vi "2_VisualizeModulePositioning.vi"(0 "Placement Monitor":T2(plugin-control), 1 "Calibrated positions of fiducials [mm]":dbl[][](array[numeric])=[[-675.4228165149058, -196.82430550413875, -11.55], [-579.8428201474238, -196.8506568257386, -11.55], [-579.816468825824, -101.27066045825673, -11.55], [-675.3964651933059, -101.24430913665685, -11.55], [-577.422820239396, -196.8513240176017, -11.55], [-481.84282387191405, -196.87767533920157, -11.55], [-481.8164725503142, -101.29767897171968, -11.55], [-577.396468917796, -101.2713276501198, -11.55], [-479.42282396388623, -196.87834253106465, -11.55], [-383.8428275964043, -196.90469385266454, -11.55], [-383.81647627480436, -101.32469748518264, -11.55], [-479.3964726422863, -101.29834616358275, -11.55], [-381.42282768837646, -196.90536104452758, -11.55], [-285.8428313208945, -196.93171236612747, -11.55], [-285.8164799992946, -101.35171599864559, -11.55], [-381.39647636677654, -101.3253646770457, -11.55], [-283.4228314128667, -196.93237955799054, -11.55], [-187.84283504538473, -196.95873087959043, -11.55], [-187.8164837237848, -101.37873451210854, -11.55], [-283.39648009126677, -101.35238319050865, -11.55], [-185.42283513735697, -196.9593980714535, -11.55], [-89.84283876987502, -196.98574939305337, -11.55], [-89.81648744827521, -101.40575302557149, -11.55], [-185.39648381575705, -101.3794017039716, -11.55], [-87.42283886184703, -196.98641658491644, -11.55], [8.157157505634814, -197.01276790651633, -11.55], [8.183508827234618, -101.43277153903443, -11.55], [-87.39648754024722, -101.40642021743454, -11.55], [10.57715741366269, -197.01343509837938, -11.55], [106.15715378114453, -197.0397864199793, -11.55], [106.18350510274433, -101.45979005249738, -11.55], [10.603508735262494, -101.4334387308975, -11.55], [108.57715368917252, -197.04045361184234, -11.55], [204.15715005665436, -197.06680493344223, -11.55], [204.18350137825416, -101.48680856596033, -11.55], [108.60350501077232, -101.46045724436046, -11.55], [206.57714996468223, -197.0674721253053, -11.55], [302.1571463321641, -197.09382344690516, -11.55], [302.1834976537639, -101.5138270794233, -11.55], [206.60350128628204, -101.4874757578234, -11.55], [304.57714624019206, -197.09449063876826, -11.55], [400.1571426076739, -197.12084196036813, -11.55], [400.1834939292737, -101.54084559288623, -11.55], [304.60349756179187, -101.51449427128635, -11.55], [402.5771425157018, -197.1215091522312, -11.55], [498.15713888318373, -197.1478604738311, -11.55], [498.18349020478354, -101.56786410634919, -11.55], [402.6034938373016, -101.5415127847493, -11.55], [500.5771387912116, -197.14852766569413, -11.55], [596.1571351586933, -197.17487898729405, -11.55], [596.1834864802931, -101.59488261981214, -11.55], [500.6034901128114, -101.56853129821225, -11.55]], 2 "XYZ .NET Refnum in":refnum<k24>, 3 "Axis Speeds":T5={"X [mm/s]"=25.0, "Y [mm/s]"=12.5, "Z [mm/s]"=5.0}, 4 "Module fiducial marker":T3(ring)=enum."[None]", 5 "N modules":i32=13, 7 "error in (no error)":errorcluster, 8 "Templates path":path=path "C:/Users/Aerotech/Documents/BNL_ThermomechanicalStave", 9 "Calibration [um/pix]":dbl=0.25, 10 "Current Build Phase":refnum<vi>, 12 "Module #":refnum<vi>, 13 "Placement tolerance [um]":dbl=10.0, 16 "Module Report":refnum<vi>) -> (22 "XYZ .NET Refnum out":refnum<k24>, 27 "error out":errorcluster)   [LabVIEW 2016]
uses:
  C:/Users/sciollalab/Documents/Brandeis-BNL/LabVIEW_Codes/BNL_ThermomechanicalStave/AerotechLibraries/Bin/Aerotech.A3200.dll
  AerotechLibraries/Bin/Aerotech.A3200.dll
  <vilib>/vision/NI_Vision_Development_Module.lvlib
panel:
  out "Offset interpreter":T1
  in  "Tab Control":enum32{"Fiducial marker", "Error reporting"}(tab)
  out "Fiducial Template":T2(plugin-control)
  out "Y offset":sgl
  out "X offset":sgl
  out "Current Stage Position":T4
  in  "Module placement loop stop":bool
  out "Module Progress Report":T6(array[cluster])
  # "VISUALIZE MODULE PLACEMENT Brandeis University - Brookhaven National Laboratory * ATLAS Phase II Inner Tracker Upgrade"
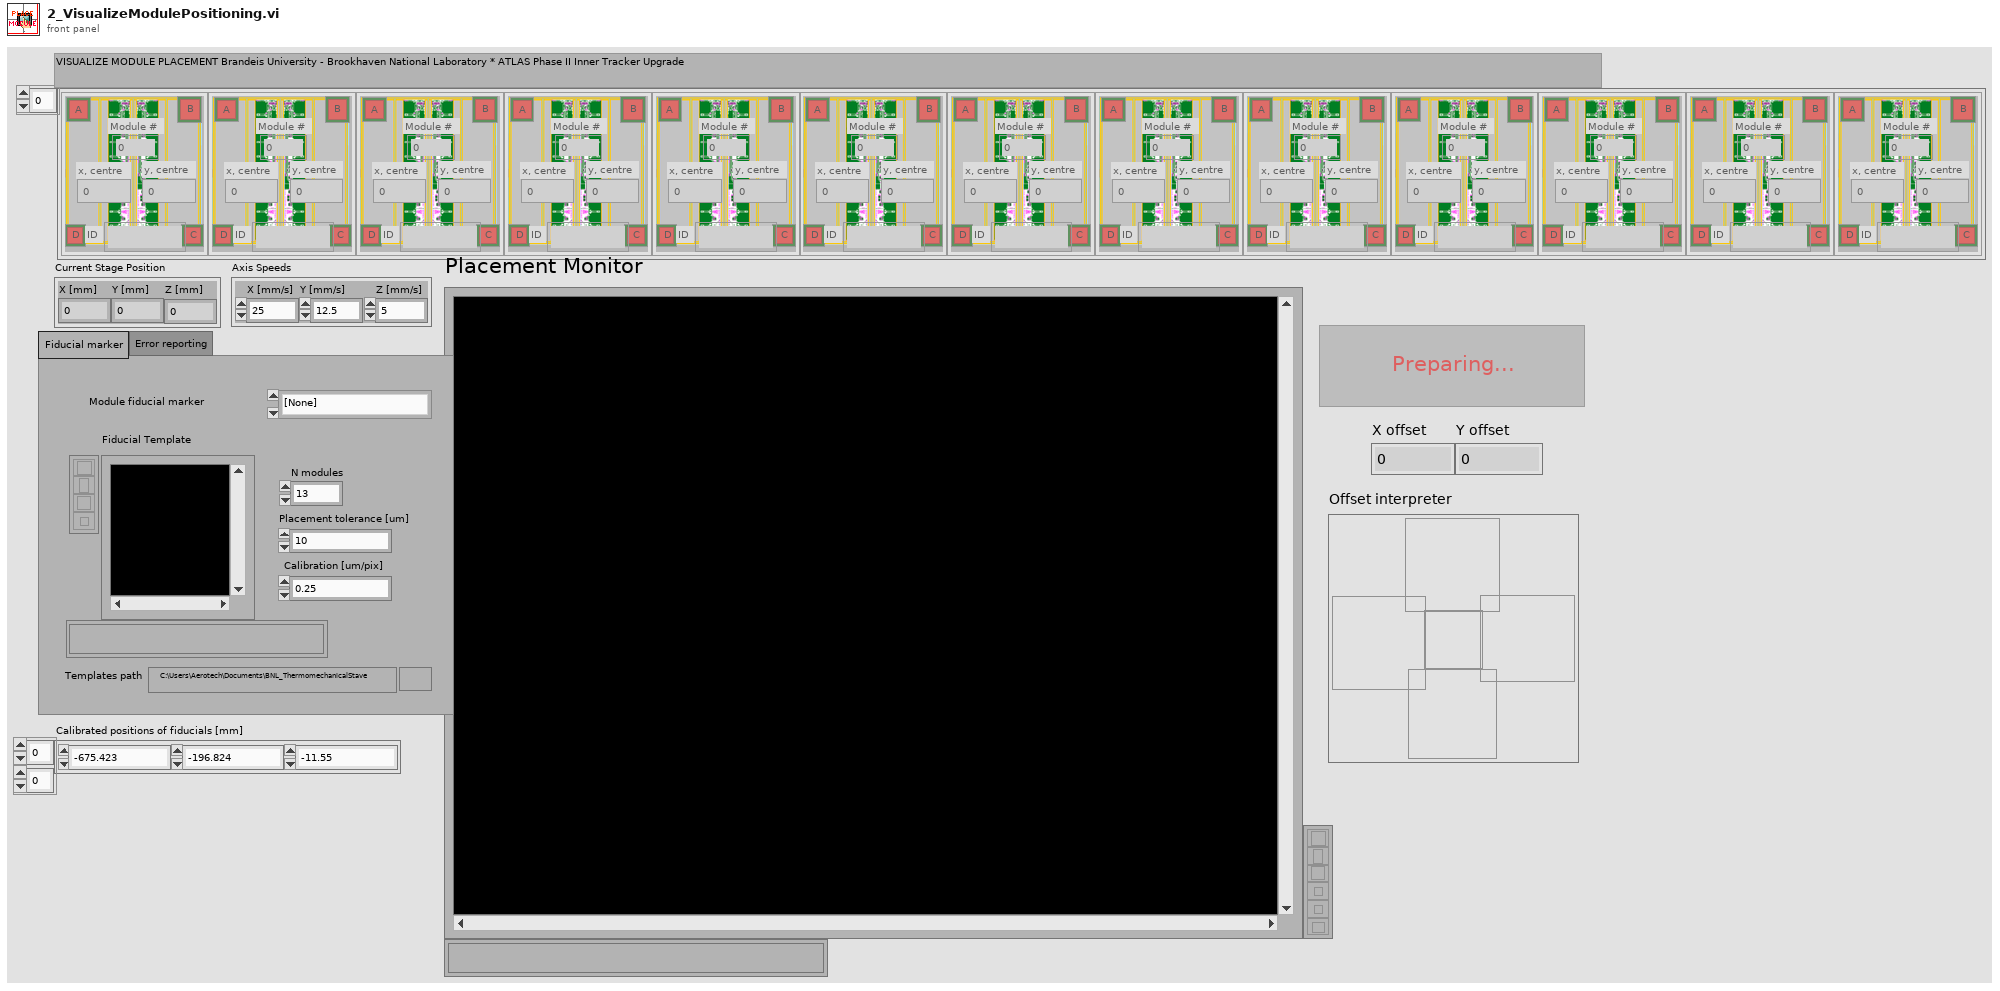
[diagram p1: front panel]
types:
  T1 = cluster{"Offset Interpreter - Right":bool, "Offset Interpreter - forward":bool, "Offset Interpreter - backward":bool, "Offset Interpreter - Left":bool, "Placement Confirmation":bool}
  T2 = typedef "IMAQ Image.ctl" = refnum<image>
  T3 = enum16{"Mark C", "Mark B", "Strip Corner", "[None]"}
  T4 = cluster{"X [mm]":dbl, "Y [mm]":dbl, "Z [mm]":dbl}
  T5 = cluster{"X [mm/s]":dbl, "Y [mm/s]":dbl, "Z [mm/s]":dbl}
  T6 = cluster{"Module #":i32, "B":bool, "A":bool, "D":bool, "C":bool, "x, centre":dbl, "y, centre":dbl, "ID":string}[]
  T7 = enum8{"Enabled", "Disabled", "Disabled and Grayed Out"}
  T8 = cluster{"Module #":i32, "B":bool, "A":bool, "D":bool, "C":bool, "x, centre":dbl, "y, centre":dbl, "Module ID":string}[]
  T9 = cluster{"Module #":i32, "B":bool, "A":bool, "D":bool, "C":bool, "x, centre":dbl, "y, centre":dbl, "Module ID":string}
  T10 = cluster{"Algorithm":i32, "Number of Matches Requested":i32, "Minimum Match Score":sgl, "SubPixel Accuracy":bool, "Rotation Angle Ranges":cluster{"Start":sgl, "End":sgl}[], "Show Search Area":bool, "Show Result":bool}
  T11 = cluster{"Module #":i32, "B":bool, "A":bool, "D":bool, "C":bool, "x, centre":dbl, "y, centre":dbl, "ID":string}
  T12 = cluster{"Final X":dbl, "Final Y":dbl, "Final Z":dbl}
  T13 = cluster{"Position":cluster{"x":sgl, "y":sgl}, "Angle":sgl, "Scale":sgl, "Score":sgl, "Bounding Box":cluster{"x":sgl, "y":sgl}[]}[]
  T14 = cluster{"Position":cluster{"x":sgl, "y":sgl}, "Angle":sgl, "Scale":sgl, "Score":sgl, "Bounding Box":cluster{"x":sgl, "y":sgl}[]}
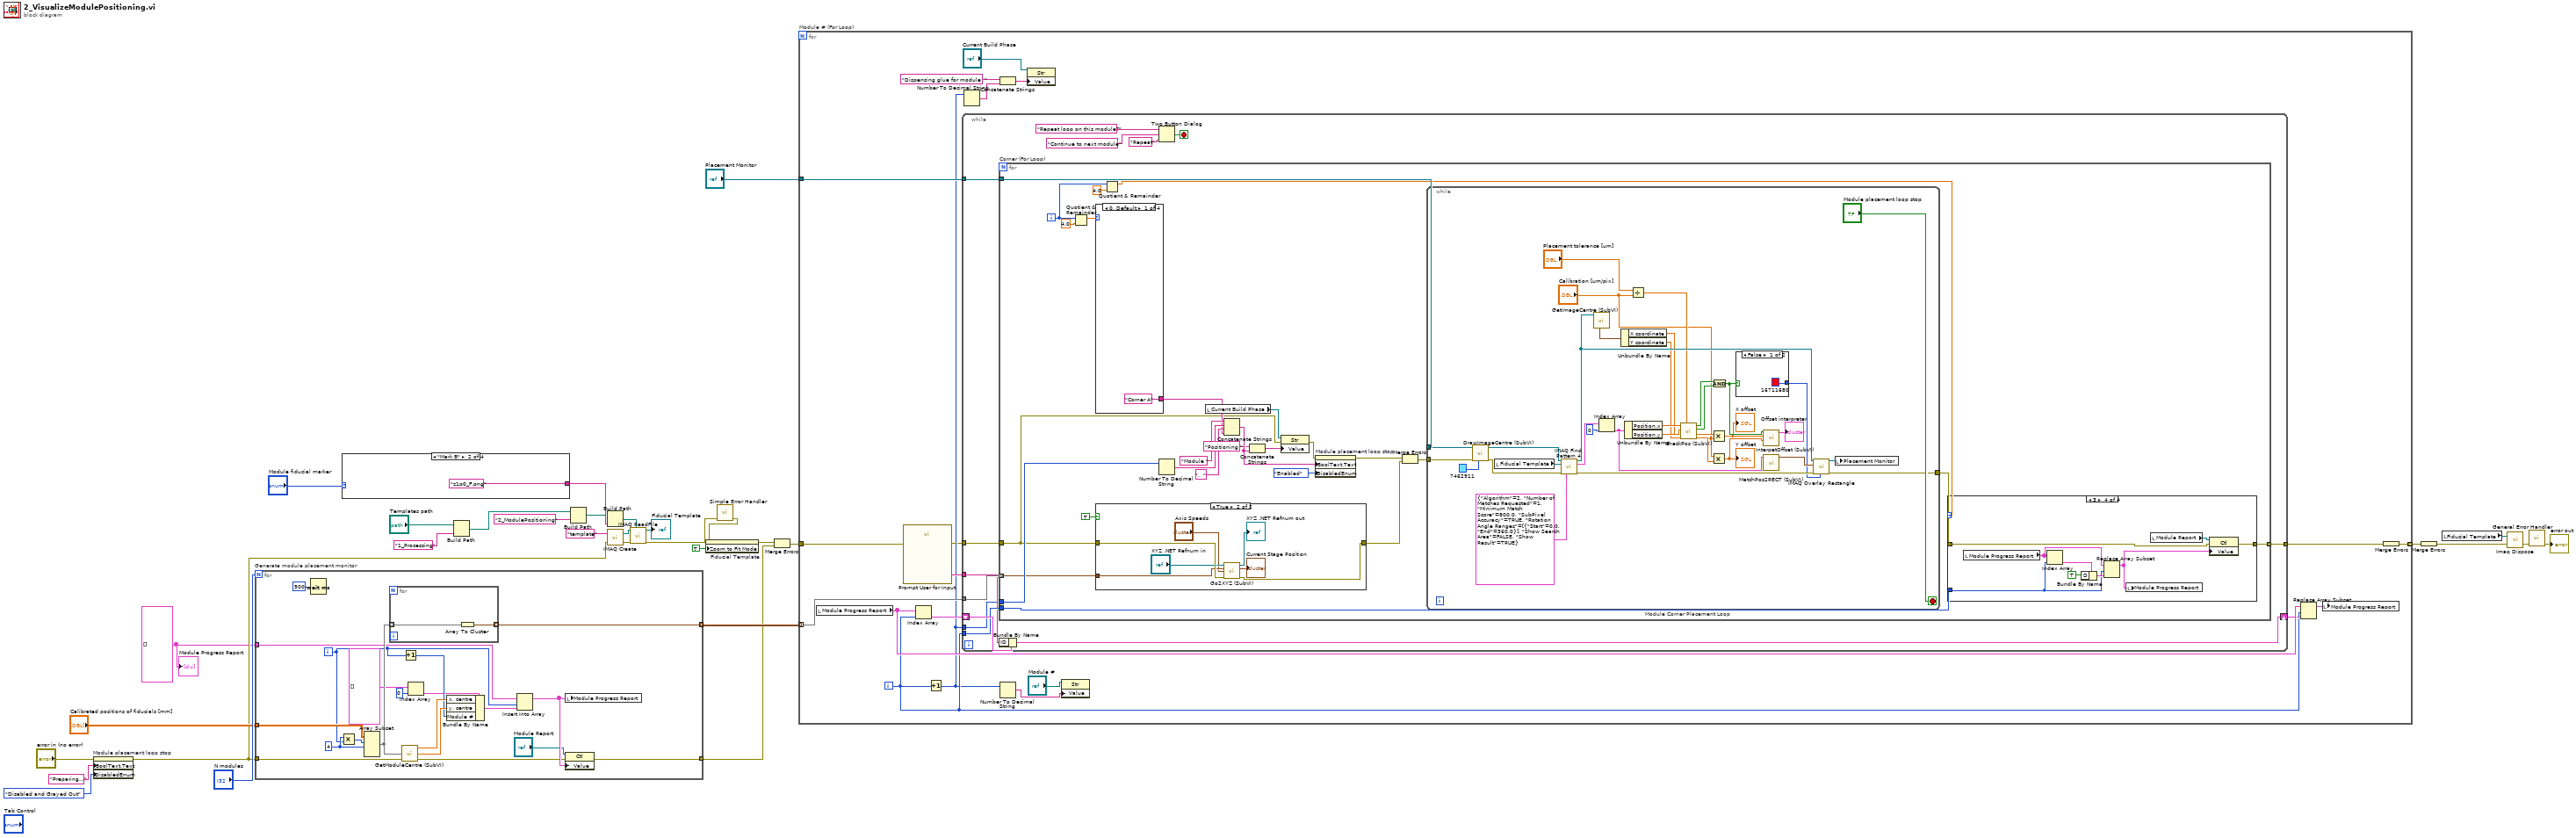
[diagram p0: block diagram]
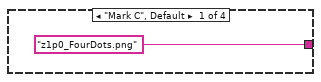
[diagram p2: hidden frame]
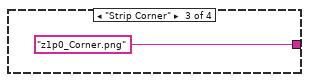
[diagram p3: hidden frame]
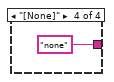
[diagram p4: hidden frame]
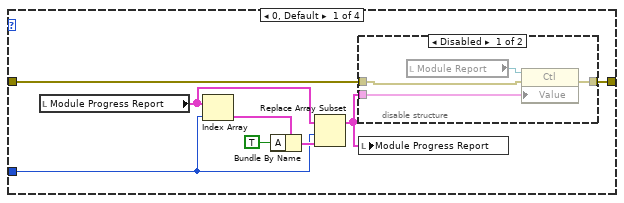
[diagram p6: hidden frame]
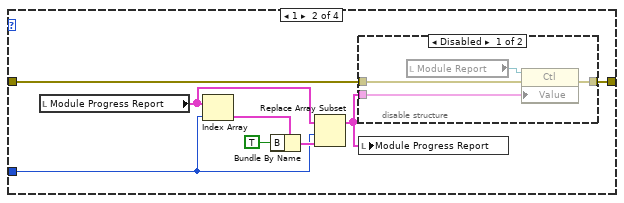
[diagram p8: hidden frame]
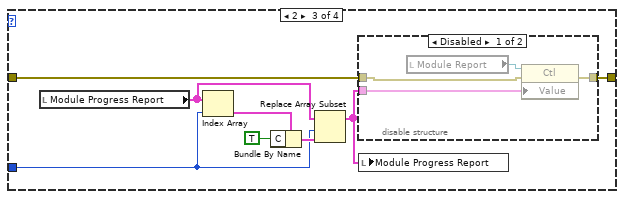
[diagram p10: hidden frame]
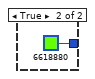
[diagram p12: hidden frame]
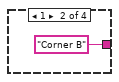
[diagram p13: hidden frame]
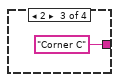
[diagram p14: hidden frame]
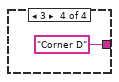
[diagram p15: hidden frame]
diagram:
  w13 = T8 [] ("Module Progress Report")
  n1 = property on="Module placement loop stop" class="Bool"(error in="error in (no error)", "BoolText.Text"="Preparing..." ("Boolean Text.Text"), "DisabledEnum"=T7."Disabled and Grayed Out" ("Disabled")) -> (error out=w18:errorcluster)  [unwired: 1 in, 1 out]
  n2 = for "Generate module placement monitor" {
    N: "N modules" -> [_]
    tunnel: "Calibrated positions of fiducials [mm]" -> [w52]
    tunnel: [w49] -> w32 mode=indexing
    tunnel: w18 -> [w39]
    tunnel: [w37] -> w25 mode=indexing
    tunnel: w13 -> [w34]
    i -> [w41]
    w50 = 4 ("x")
    n3 = Wait (ms)(milliseconds to wait=u32 500) -> ()  [unwired: 1 out]
    n4 = Multiply(x=w50, y=w41) -> (x*y=w51:i32)
    n5 = Array Subset(array=w52, index (row)=w51, length (row)=w50) -> (w48:dbl[][])  [unwired: 2 in]
    n6 = for {
      tunnel: w48 -> [w53] mode=indexing
      tunnel: [w54] -> w49 mode=indexing
      n7 = Array To Cluster(array=w53) -> (cluster=w54:cluster{"[0]":dbl, "[1]":dbl, "[2]":dbl})
    }
    n8 = call "GetModuleCentre (SubVI).vi"("error in (no error)"=w39, "4x3 Array of Fiducial Coordinates"=w48) -> ("error out"=w38:errorcluster, "y, centre"=w46:dbl, "x, centre"=w47:dbl)  [unwired: 1 in]
    n9 = Increment(x=w41) -> (x+1=w45:i32)
    n10 = Index Array(array=T8 [] ("Module Progress Report"), index=0) -> (element=w42:T9)
    n11 = Bundle By Name(cluster=w42, "x, centre"=w47, "y, centre"=w46, "Module #"=w45) -> (w36:T9)
    n12 = Insert Into Array(array=w34, index=w41, new element=w36) -> (w40:T8)
    n13 = local write "Module Progress Report"(w40) -> ()
    n14 = property class="Ctl"(reference="Module Report", error in=w38, "Value"=w40) -> (error out=w37:errorcluster)  [unwired: 1 out]
  }
  n15 = case shown="\"Mark B\"" "Module fiducial marker" {
    tunnel: ["z1p0_FourDots.png" ("name or relative path") "z1p0_F.png" ("name or relative path") "z1p0_Corner.png" ("name or relative path") "none" ("name or relative path")] -> w21
    frame "Mark C", Default {
    }
    frame "Mark B" {
    }
    frame "Strip Corner" {
    }
    frame "[None]" {
    }
  }
  n16 = Build Path(base path="Templates path", name or relative path="1_Processing") -> (appended path=w8:path)
  n17 = Build Path(base path=w8, name or relative path="2_ModulePositioning") -> (appended path=w20:path)
  n18 = Build Path(base path=w20, name or relative path=w21) -> (appended path=w7:path)
  n19 = call "IMAQ Create"("Image Name"="template", "error in (no error)"=w18) -> ("New Image"=w6:T2, "error out"=w5:errorcluster)  [unwired: 3 in]
  n20 = call "IMAQ ReadFile"("File Path"=w7, "error in (no error)"=w5, "Image"=w6) -> ("error out"=w2:errorcluster, "Image Out"=→"Fiducial Template":T2)  [unwired: 4 in, 3 out]
  n21 = call <vilib>:"Simple Error Handler.vi"("error in (no error)"=w2) -> ("error out"=w1:errorcluster)  [unwired: 4 in, 4 out]
  n22 = property on="Fiducial Template" class="ImageControl"(error in=w1, "Zoom to Fit Mode"=TRUE) -> (error out=w26:errorcluster)  [unwired: 1 in, 1 out]
  n23 = Merge Errors(w26, w25) -> (w24:errorcluster)
  n24 = for "Module # (For Loop)" {
    tunnel: "Placement Monitor" -> [w77]
    tunnel: w24 -> [w62]
    tunnel: w32 -> [w76] mode=indexing
    tunnel: [w74] -> w31 mode=indexing
    i -> [w69]
    n25 = local read "Module Progress Report"() -> (w73:T6)
    n26 = call "Prompt User for Input"("error in (no error)"=w62) -> ("Module ID"=w68:string, "error out"=w61:errorcluster)  [unwired: 16 in, 1 out]
    n27 = Index Array(array=w73, index=w69) -> (element=w72:T11)
    n28 = Increment(x=w69) -> (x+1=w63:i32)
    n29 = while {
      tunnel: w77 -> [w90]
      tunnel: w76 -> [w89]
      tunnel: [w88] -> w75
      tunnel: w69 -> [w85]
      tunnel: w68 -> [w84]
      tunnel: w63 -> [w83]
      tunnel: w61 -> [w82]
      shift-right: [w86] -> w71
      shift-left: w72 -> [w87]
      stop <- w81 stop-if-true
      n30 = for "Corner (For Loop)" {
        tunnel: w90 -> [w116]
        tunnel: w82 -> [w97]
        tunnel: w83 -> [w112]
        tunnel: w89 -> [w108] mode=indexing
        tunnel: w85 -> [w107]
        tunnel: [w95] -> w88 mode=indexing
        i -> [w106]
        n31 = Quotient & Remainder(x=w106, y=4.0) -> (x-y*floor(x/y)=w109:dbl)  [unwired: 1 out]
        n32 = case shown="0, Default" w109 {
          tunnel: ["Corner A" "Corner B" "Corner C" "Corner D"] -> w111
          frame 0, Default {
          }
          frame 1 {
          }
          frame 2 {
          }
          frame 3 {
          }
        }
        n33 = case shown="True" TRUE {
          tunnel: w97 -> [w117 w124]
          tunnel: [w117 w122] -> w93
          tunnel: w108 -> [_ w123]
          frame False {
            # "Temporarily skip corners C and D"
          }
          frame True {
            n34 = call "Go2XYZ (SubVI).vi"(".NET Refnum in"="XYZ .NET Refnum in", "Go to Coordinates"=w123, "Axis Speeds"="Axis Speeds", "error in (no error)"=w124) -> (".NET Refnum out"=→"XYZ .NET Refnum out":refnum<k24>, "Final Position"=→"Current Stage Position":T12, "error out"=w122:errorcluster)  [unwired: 7 in, 2 out]
          }
        }
        n35 = Quotient & Remainder(x=w106, y=4.0) -> (x-y*floor(x/y)=w100:dbl)  [unwired: 1 out]
        n36 = Number To Decimal String(number=w112) -> (decimal integer string=w115:string)  [unwired: 1 in]
        n37 = local read "Current Build Phase"() -> (w103:refnum<vi>)
        n38 = Concatenate Strings("Module " ("string"), w115, ",  " ("string"), w111) -> (w104:string)
        n39 = Concatenate Strings("Positioning " ("string"), w104) -> (w101:string)
        n40 = property class="Str"(reference=w103, error in=w97, "Value"=w101) -> (error out=w98:errorcluster)  [unwired: 1 out]
        n41 = property on="Module placement loop stop" class="Bool"(error in=w98, "BoolText.Text"=w104, "DisabledEnum"=T7."Enabled" ("Disabled")) -> (error out=w94:errorcluster)  [unwired: 1 in, 1 out]
        n42 = Merge Errors(w94, w93) -> (w92:errorcluster)
        n43 = while "Module Corner Placement Loop" {
          tunnel: w116 -> [w202]
          tunnel: w92 -> [w201]
          tunnel: [w199] -> w96
          stop <- "Module placement loop stop" stop-if-true
          n44 = call "DrawImageCentre (SubVI).vi"("Axis colour"=u32 7462911, "error in (no error)"=w201, "Refnum in"=w202) -> ("error out"=w179:errorcluster, "Refnum out"=w180:T2)  [unwired: 7 in]
          n45 = local read "Fiducial Template"() -> (w197:T2)
          n46 = call "IMAQ Find Pattern 4"("Image"=w180, "Template"=w197, "error in"=w179, "Settings"=T10 {"Algorithm"=2, "Number of Matches Requested"=1, "Minimum Match Score"=800.0, "SubPixel Accuracy"=TRUE, "Rotation Angle Ranges"=[{"Start"=0.0, "End"=360.0}], "Show Search Area"=FALSE, "Show Result"=TRUE}) -> ("Image Out"=w188:T2, "Matches (pixel)"=w195:T13, "error out"=w193:errorcluster)  [unwired: 5 in, 4 out]
          n47 = call "GetImageCentre (SubVI).vi"("Image in \n(refnum)"=w188) -> ("Centre Point"=w187:cluster{"X coordinate":dbl, "Y coordinate":dbl})  [unwired: 4 in, 4 out]
          n48 = Index Array(array=w195, index=0) -> (element=w183:T14)
          n49 = Unbundle By Name(w187) -> ("X coordinate"=w186:dbl, "Y coordinate"=w185:dbl)
          n50 = Unbundle By Name(w183) -> ("Position.x"=w192:sgl, "Position.y"=w191:sgl)
          n51 = Divide(x="Placement tolerance [um]", y="Calibration [um/pix]") -> (x/y=w177:dbl)
          n52 = call "CheckPos (SubVI).vi"("x"=w192, "y"=w191, "true x"=w186, "true y"=w185, "variation tolerance"=w177) -> ("pass x coordinate"=w190:bool, "pass y coordinate"=w189:bool, "delta X"=w182:sgl, "delta Y"=w181:sgl)  [unwired: 2 in]
          n53 = Multiply(x=w182, y="Calibration [um/pix]") -> (x*y=w172:dbl)
          "X offset" <- w172
          n54 = Multiply(x="Calibration [um/pix]", y=w181) -> (x*y=w171:dbl)
          "Y offset" <- w171
          n55 = And(x=w190, y=w189) -> (x .and. y?=w173:bool)
          n56 = case shown="False" w173 {
            tunnel: [u32 16711680 ("Color") u32 6618880 ("Color")] -> w184
            frame False {
            }
            frame True {
            }
          }
          n57 = call "InterpetOffset (SubVI).vi"("Y offset"=w171, "X offset"=w172, "Good position"=w173) -> ("Offset interpreter"=→"Offset interpreter":T1)  [unwired: 8 in]
          n58 = call "MatchPos2RECT (SubVI).vi"("Match element"=w183) -> ("Rectangle"=w196:cluster{"x":sgl, "y":sgl, dbl, dbl})  [unwired: 10 in]
          n59 = call "IMAQ Overlay Rectangle"("Color"=w184, "error in (no error)"=w193, "Rectangle"=w196, "Image"=w188) -> ("error out"=w199:errorcluster, "Image Out"=w176:T2)  [unwired: 6 in]
          n60 = local write "Placement Monitor"(w176) -> ()
        }
        n61 = case shown="3" w100 {
          tunnel: w107 -> [w129 w140 w152 w165]
          tunnel: w96 -> [w126 w138 w150 w163]
          tunnel: [w125 w137 w149 w162] -> w95
          frame 0, Default {
            n62 = local read "Module Progress Report"() -> (w130:T6)
            n63 = Index Array(array=w130, index=w129) -> (element=w128:T11)
            n64 = Bundle By Name(cluster=w128, "A"=TRUE) -> (w131:T11)
            n65 = Replace Array Subset(array=w130, new element=w131, index=w129) -> (w127:T6)
            n66 = disable-structure shown="Disabled" {
              disable-tunnel: w127 -> [w135 _]
              disable-tunnel: w126 -> [w134 _]
              disable-tunnel: [w133 _] -> w125
              frame Disabled {
                n67 = local read "Module Report"() -> (w136:refnum<vi>)
                n68 = property class="Ctl"(reference=w136, error in=w134, "Value"=w135) -> (error out=w133:errorcluster)  [unwired: 1 out]
              }
              frame Enabled {
              }
            }
            n69 = local write "Module Progress Report"(w127) -> ()
          }
          frame 1 {
            n70 = local read "Module Progress Report"() -> (w142:T6)
            n71 = Index Array(array=w142, index=w140) -> (element=w141:T11)
            n72 = Bundle By Name(cluster=w141, "B"=TRUE ("A")) -> (w143:T11)
            n73 = Replace Array Subset(array=w142, new element=w143, index=w140) -> (w139:T6)
            n74 = disable-structure shown="Disabled" {
              disable-tunnel: w139 -> [w147 _]
              disable-tunnel: w138 -> [w146 _]
              disable-tunnel: [w145 _] -> w137
              frame Disabled {
                n75 = local read "Module Report"() -> (w148:refnum<vi>)
                n76 = property class="Ctl"(reference=w148, error in=w146, "Value"=w147) -> (error out=w145:errorcluster)  [unwired: 1 out]
              }
              frame Enabled {
              }
            }
            n77 = local write "Module Progress Report"(w139) -> ()
          }
          frame 2 {
            n78 = local read "Module Progress Report"() -> (w154:T6)
            n79 = Index Array(array=w154, index=w152) -> (element=w153:T11)
            n80 = Bundle By Name(cluster=w153, "C"=TRUE ("A")) -> (w155:T11)
            n81 = Replace Array Subset(array=w154, new element=w155, index=w152) -> (w151:T6)
            n82 = disable-structure shown="Disabled" {
              disable-tunnel: w151 -> [w159 _]
              disable-tunnel: w150 -> [w158 _]
              disable-tunnel: [w157 _] -> w149
              frame Disabled {
                n83 = local read "Module Report"() -> (w160:refnum<vi>)
                n84 = property class="Ctl"(reference=w160, error in=w158, "Value"=w159) -> (error out=w157:errorcluster)  [unwired: 1 out]
              }
              frame Enabled {
              }
            }
            n85 = local write "Module Progress Report"(w151) -> ()
          }
          frame 3 {
            n86 = local read "Module Progress Report"() -> (w167:T6)
            n87 = Index Array(array=w167, index=w165) -> (element=w166:T11)
            n88 = Bundle By Name(cluster=w166, "D"=TRUE ("A")) -> (w168:T11)
            n89 = Replace Array Subset(array=w167, new element=w168, index=w165) -> (w164:T6)
            n90 = local write "Module Progress Report"(w164) -> ()
            n91 = local read "Module Report"() -> (w161:refnum<vi>)
            n92 = property class="Ctl"(reference=w161, error in=w163, "Value"=w164) -> (error out=w162:errorcluster)  [unwired: 1 out]
          }
        }
      }
      n93 = Bundle By Name(cluster=w87, "ID"=w84) -> (w86:T11)
      n94 = Two Button Dialog(message="Repeat loop on this module?", 1:"Repeat" ("F button name (\"Cancel\")"), 2:"Continue to next module" ("T button name (\"OK\")")) -> (T button?=w81:bool)
    }
    n95 = Number To Decimal String(number=w63) -> (decimal integer string=w64:string)  [unwired: 1 in]
    n96 = Concatenate Strings("Dispensing glue for module  " ("string"), w64) -> (w66:string)
    n97 = Number To Decimal String(number=w63) -> (decimal integer string=w59:string)  [unwired: 1 in]
    n98 = property class="Str"(reference="Current Build Phase", "Value"=w66) -> ()  [unwired: 1 in, 2 out]
    n99 = property class="Str"(reference="Module #", "Value"=w59) -> ()  [unwired: 1 in, 2 out]
    n100 = Replace Array Subset(array=w73, new element=w71, index=w69) -> (w70:T6)
    n101 = local write "Module Progress Report"(w70) -> ()
    n102 = Merge Errors(w75) -> (w74:errorcluster)
  }
  n103 = Merge Errors(w31) -> (w28:errorcluster)
  n104 = local read "Fiducial Template"() -> (w30:T2)
  n105 = call "Imaq Dispose"("Image"=w30, "error in (no error)"=w28) -> ("error out"=w29:errorcluster)  [unwired: 4 in]
  n106 = call <vilib>:"General Error Handler.vi"("error in (no error)"=w29) -> ("error out"=→"error out":errorcluster)  [unwired: 10 in, 4 out]
  "Module Progress Report" <- w13
